vi "Untitled 1.vi"(4 "User Parameter":variant, 5 "Event Data":cluster{"uiMsg":refnum<k7>, "cancel":bool}, 6 "Control Ref":refnum<k7>, 7 "Event Common Data":T1) -> (1 "Event Data Out":cluster{"cancel":bool})   [LabVIEW 2018]
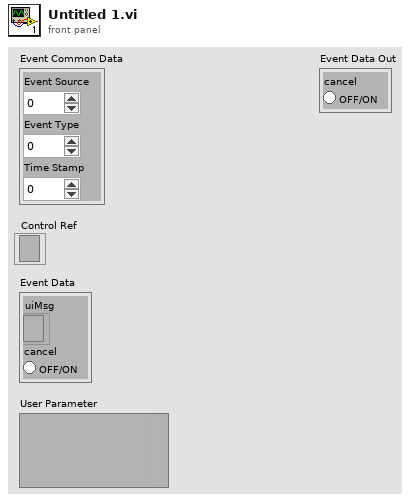
[diagram p1: front panel]
types:
  T1 = cluster{"Event Source":i32, "Event Type":u32, "Time Stamp":u32}
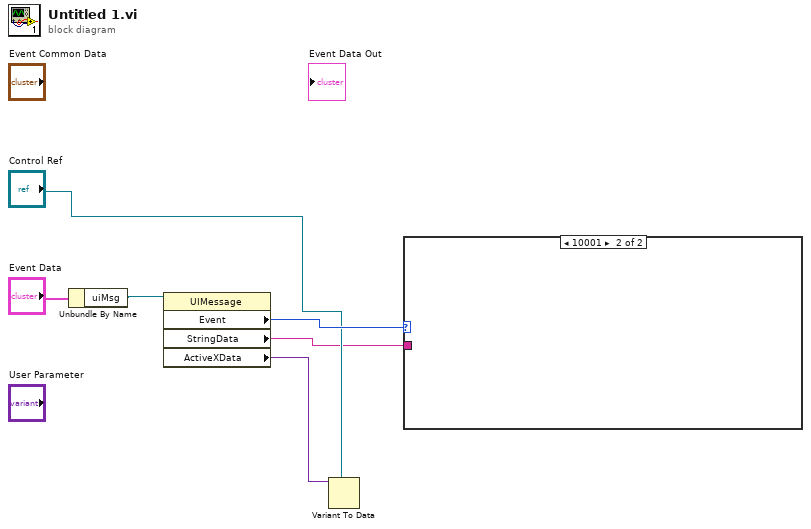
[diagram p0: block diagram]
diagram:
  n1 = Unbundle By Name("Event Data") -> ("uiMsg"=w5:refnum<k7>)
  n2 = property class="UIMessage"(reference=w5) -> ("Event"=w4:i32, "StringData"=w1:string, "ActiveXData"=w3:variant)  [unwired: 1 in, 2 out]
  n3 = Variant To Data(type="Control Ref", Variant=w3) -> ()  [unwired: 1 in, 2 out]
  n4 = case shown="10001" w4 {
    tunnel: w1 -> [_ _]
    frame 0, Default {
    }
    frame 10001 {
    }
  }
